vi "create_new.vi"(6 "Optional":T1, 9 "Labels":refnum<class "labels.lvclass">, 10 "Properties":refnum<class "properties.lvclass">) -> (3 "New Target":refnum<class "target.lvclass">)   [LabVIEW 2020, in "datasources.lvlib" / "target.lvclass"]
uses:
  target.lvclass
  nominal types/properties/properties.lvclass
  nominal types/labels/labels.lvclass
  dataset/dataset.lvclass
  nominal types/channelConfig/channelConfig.lvclass
  target.lvclass/target.ctl
  properties.set.vi
  labels.set.vi
  dataset.set.vi
  channelConfig.set.vi
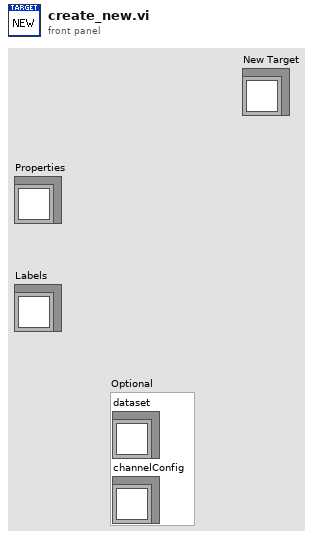
[diagram p1: front panel]
types:
  T1 = cluster{"dataset":refnum<class "dataset.lvclass">, "channelConfig":refnum<class "channelConfig.lvclass">}
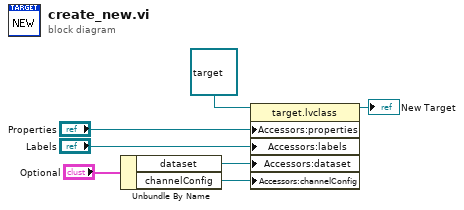
[diagram p0: block diagram]
diagram:
  n1 = Unbundle By Name("Optional") -> ("dataset"=w3:refnum<class "dataset.lvclass">, "channelConfig"=w2:refnum<class "channelConfig.lvclass">)
  n2 = property class="target.lvclass"(reference=refnum<class "target.lvclass"> refnum ("Target"), "Accessors:properties"="Properties", "Accessors:labels"="Labels", "Accessors:dataset"=w3, "Accessors:channelConfig"=w2) -> (reference out=→"New Target":refnum<class "target.lvclass">)  [unwired: 1 in, 1 out]
